vi "Stop Tx.vi"(8 "error in (no error)":errorcluster, 11 "channel":i32) -> (0 "error out":errorcluster, 3 "function return":bool)   [LabVIEW 2014, in "QCA_DUT_Func.lvlib"]
doc: "DLL_QMSL_AEROFLEX bool _stdcall StopTx(int channel);"
uses:
  QCA_DUT_Func.lvlib
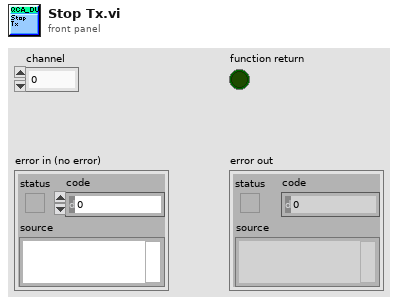
[diagram p1: front panel]
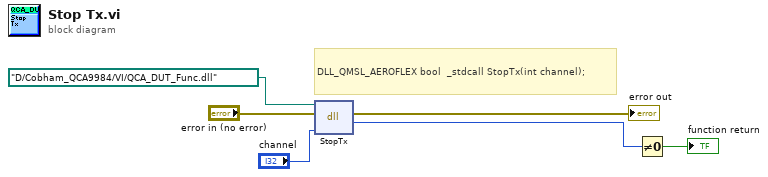
[diagram p0: block diagram]
diagram:
  # "DLL_QMSL_AEROFLEX bool  _stdcall StopTx(int channel);"
  n1 = dll-call lib="D:/Cobham_QCA9984/VI/QCA_DUT_Func.dll" fn="StopTx"(path in=path "D:/Cobham_QCA9984/VI/QCA_DUT_Func.dll", error in="error in (no error)", "channel"="channel") -> (error out=→"error out":errorcluster, "return type"=w5:u8)  [unwired: 2 in, 1 out]
  n2 = Not Equal To 0?(x=w5) -> (x != 0?=→"function return":bool)
